vi "Do.vi"(8 "error in":errorcluster, 10 "Actor in":refnum<class "Actor.lvclass">, 11 "Change PAS Fmod MSG":refnum<class "Forward Command MSG.lvclass">) -> (0 "error out":errorcluster, 2 "Actor out":refnum<class "Actor.lvclass">)   [LabVIEW 2017, in "Controller.lvlib" / "Forward Command MSG.lvclass"]
doc: "(<B>Filename</B>: Actor Framework.lvlib:Message.lvclass:Do.vi)\n\nDefines what a message does when it is received by an actor. Generally, a message instructs an actor to invoke one of its methods. By default, this method does nothing. A child class must override it to define behavior. Create a child class by using the Actor Framework Message Maker dialog box."
uses:
  Forward Command MSG.lvclass
  <vilib>/ActorFramework/Actor/Actor.lvclass
  Forward Command MSG.lvclass/Forward Command MSG.ctl
  <vilib>/MSR Consulting, LLC/General Reuse/SuperActor/SuperActor.lvclass
  C:/Program Files (x86)/National Instruments/LabVIEW 2017/vi.lib/ActorFramework/Actor/Actor.lvclass
  <vilib>/MSR Consulting, LLC/General Reuse/SuperActor/SuperActor.lvclass/SuperActor.ctl
  <vilib>/ActorFramework/Message Enqueuer/Message Enqueuer.lvclass
  Support/Send Command/Send Command MSG.lvclass
  C:/Program Files (x86)/National Instruments/LabVIEW 2017/vi.lib/ActorFramework/Message/Message.lvclass
  Support/Send Command/Send Command MSG.lvclass/Send Command MSG.ctl
  <vilib>/ActorFramework/Message Enqueuer/Message Enqueuer.lvclass/Message Enqueuer.ctl
  <vilib>/MSR Consulting, LLC/General Reuse/SuperActor/Read EnqueuerMap.vi
  <vilib>/MSR Consulting, LLC/General Reuse/SuperActor/Read Log Session.vi
  Support/Send Command/Write CMD.vi
  <vilib>/ActorFramework/Message Priority Queue/Priority Enqueue.vi
  <vilib>/MSR Consulting, LLC/General Reuse/Session APIs/_Session Fwk/Session - Root.lvclass
  <vilib>/MSR Consulting, LLC/General Reuse/Session APIs/Session Log/System Log.lvclass
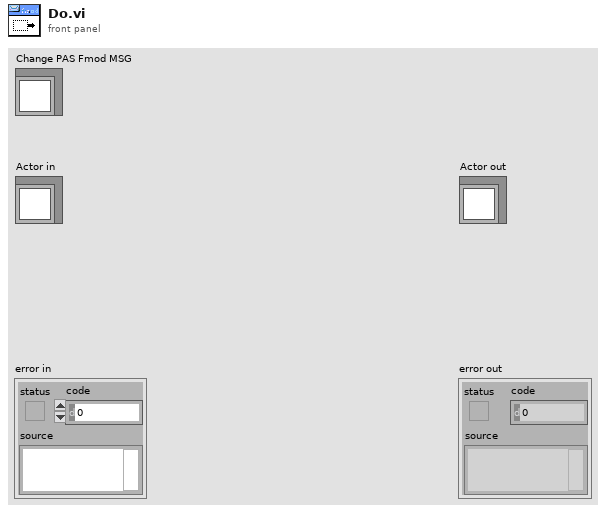
[diagram p1: front panel]
types:
  T1 = typedef "Session - Root.lvclass/Session Handle.ctl" = refnum<data-value>
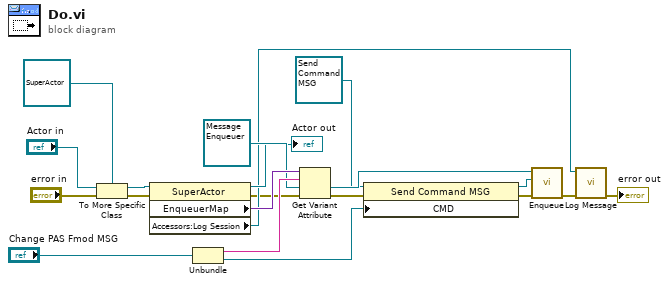
[diagram p0: block diagram]
diagram:
  n1 = To More Specific Class(target class=refnum<class "SuperActor.lvclass"> refnum ("SuperActor.lvlib:SuperActor"), reference="Actor in", error in="error in") -> (specific class reference=w17:refnum<class "SuperActor.lvclass">, error out=w18:errorcluster)
  n2 = property class="SuperActor"(reference=w17, error in=w18) -> (reference out=→"Actor out":refnum<class "SuperActor.lvclass">, error out=w4:errorcluster, "EnqueuerMap"=w16:variant, "Accessors:Log Session"=w6:T1)
  n3 = Unbundle("Change PAS Fmod MSG") -> (w14:string, w10:refnum<class "Command.lvclass">)
  n4 = Get Variant Attribute(Variant=w16, name=w14, default value (empty Variant)=refnum<class "Message Enqueuer.lvclass"> refnum ("Message Enqueuer in"), error in=w4) -> (value=w12:refnum<class "Message Enqueuer.lvclass">, error out=w3:errorcluster)  [unwired: 2 out]
  n5 = property class="Send Command MSG"(reference=refnum<class "Send Command MSG.lvclass"> refnum ("Send Command MSG"), error in=w3, "CMD"=w10) -> (reference out=w9:refnum<class "Send Command MSG.lvclass">, error out=w2:errorcluster)
  n6 = call <vilib>:"Enqueue.vi"("error in (no error)"=w2, "Message"=w9, "Message Enqueuer in"=w12) -> ("error out"=w1:errorcluster)  [unwired: 7 in, 1 out]
  n7 = call <vilib>:"Log Message.vi"("error in"=w1, "session in"=w6) -> ("error out"=→"error out":errorcluster)  [unwired: 8 in, 1 out]
